vi "JPL Potentiometer PID (SubVI).vi"(4 "refnum name":string, 5 "Potentiometer Config":cluster{"Elevator Height":dbl, "Offset":dbl}, 6 "PID Settings":T2, 7 "PID Limits":cluster{"Upper Limit":dbl, "Lower Limit":dbl}) -> (0 "Potentiometer Status":T1, 3 "output":dbl)   [LabVIEW 2014]
uses:
  <vilib>/addons/control/pid/pid.llb/PID (DBL).vi
  <vilib>/addons/control/pid/NI_PID_pid.lvlib
panel:
  out "Potentiometer Voltage Chart":dbl(graph)
  out "PID Output Chart":dbl(graph)
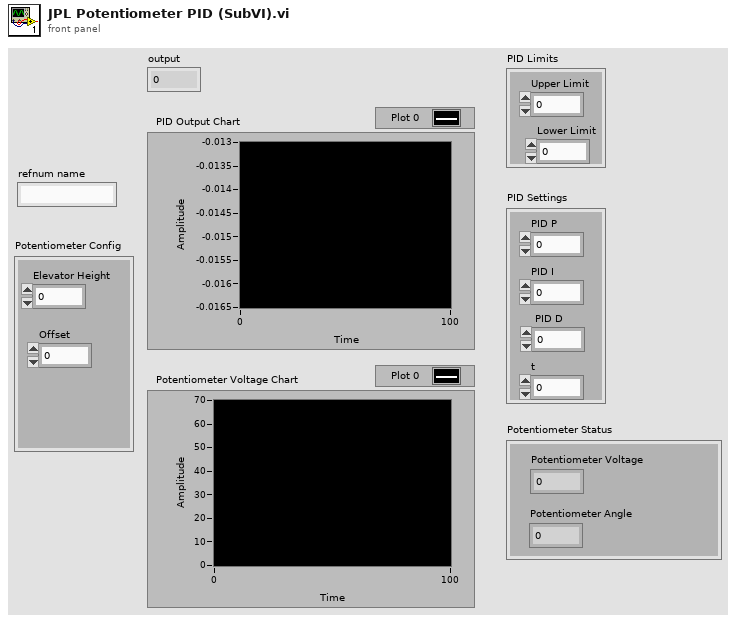
[diagram p1: front panel]
types:
  T1 = cluster{"Potentiometer Voltage":dbl, "Potentiometer Angle":dbl}
  T2 = cluster{"PID P":dbl, "PID I":dbl, " PID D":dbl, "t":dbl}
  T3 = typedef "WPI_PotentiometerDevRef.ctl" = cluster{"DevStatus":errorcluster, "Controller":T4, "Analog Channel":T5, "Invert Output":bool}
  T4 = typedef "FPGA_TypedefAnalogModule.ctl" = enum16{"Controller 1"}
  T5 = typedef "FPGA_AIChannel.ctl" = enum8{"AI 0", "AI 1", "AI 2", "AI 3", "AI MXP 0", "AI MXP 1", "AI MXP 2", "AI MXP 3", "Invalid"}
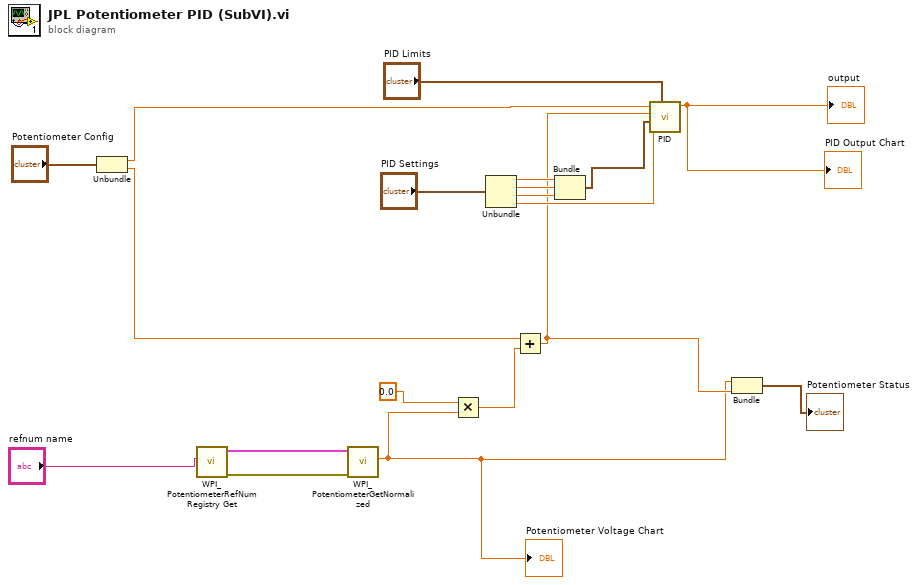
[diagram p0: block diagram]
diagram:
  n1 = Unbundle("Potentiometer Config") -> ("Elevator Height"=w6:dbl, "Offset"=w7:dbl)
  n2 = call <vilib>:"WPI_PotentiometerRefNum Registry Get.vi"("refnum name"="refnum name") -> ("error out"=w4:errorcluster, "PotDevRef"=w5:T3)  [unwired: 9 in]
  n3 = call <vilib>:"WPI_PotentiometerGetNormalized.vi"("error in"=w4, "PotDevRef"=w5) -> ("Normalized Value"=w1:dbl)  [unwired: 7 in, 2 out]
  "Potentiometer Voltage Chart" <- w1
  n4 = Multiply(x=0.0, y=w1) -> (x*y=w2:dbl)
  n5 = Unbundle("PID Settings") -> ("PID P"=w15:dbl, "PID I"=w14:dbl, "PID D"=w13:dbl, "t"=w12:dbl)
  n6 = Add(x=w7, y=w2) -> (x+y=w9:dbl)
  n7 = Bundle("PID P"=w15, "PID I"=w14, "PID D"=w13) -> (w11:cluster{"PID P":dbl, "PID I":dbl, " PID D":dbl})  [unwired: 1 in]
  n8 = call-poly <vilib>:"PID.vi"("output range"="PID Limits", "dt (s)"=w12, "PID gains"=w11, "process variable"=w9, "setpoint"=w6) -> ("output"=→"PID Output Chart" →"output":dbl)  [unwired: 5 in, 1 out]
  n9 = Bundle("Normalized Value"=w1, w9) -> (→"Potentiometer Status":cluster{"Normalized Value":dbl, dbl})  [unwired: 1 in]
